vi "Array Manipulation.vi"() -> ()   [LabVIEW 2015]
doc: "This VI shows how different array functions can be used to manipulate data. There are also examples showing how we can use the Polymorphic functionality built into LabVIEW to easily modify the data in an array. \n\nExamine the different cases and read the comments on the block diagram for more details"
uses:
  <vilib>/measure/NI_MABase.lvlib
panel:
  in  "Stop Button":bool
  in  "Tab Control":T1(tab)
  out "Concatenated Data Array":dbl[](array[numeric])
  out "Concatenated Data":dbl[](graph)
  in  "Subtract?":bool
  out "Add or Subtract Data Array":dbl[](array[numeric])
  out "Add or Subtract Data":dbl[](graph)
  in  "Select Channel":u16(ring) items=["Channel 0", "Channel 1"]
  out "Single Channel of Data Array":dbl[](array[numeric])
  out "Single Channel of Data":dbl[](graph)
  out "Size of Array":i32
  in  "Offset":dbl(slide)=-8.326672684688674e-17 scale=-5.0..5.0
  out "Waveform Data":waveform(dbl)[](graph)
  out "Data Channel Array":dbl[][](array[numeric])
  in  "Channel 1 Offset":dbl(slide)=-8.326672684688674e-17 scale=-5.0..5.0
  out "All Data Channel":dbl[][](graph)
  out "Size of Array":i32[](array[numeric])
  out "Subset Data Array":dbl[][](array[numeric])
  in  "Start Value":i32(slide)=10 scale=0.0..1000.0
  out "Subset Data":dbl[][](graph)
  in  "Length":i32(slide)=1000 scale=0.0..1000.0
  # "Rows"
  # "Columns"
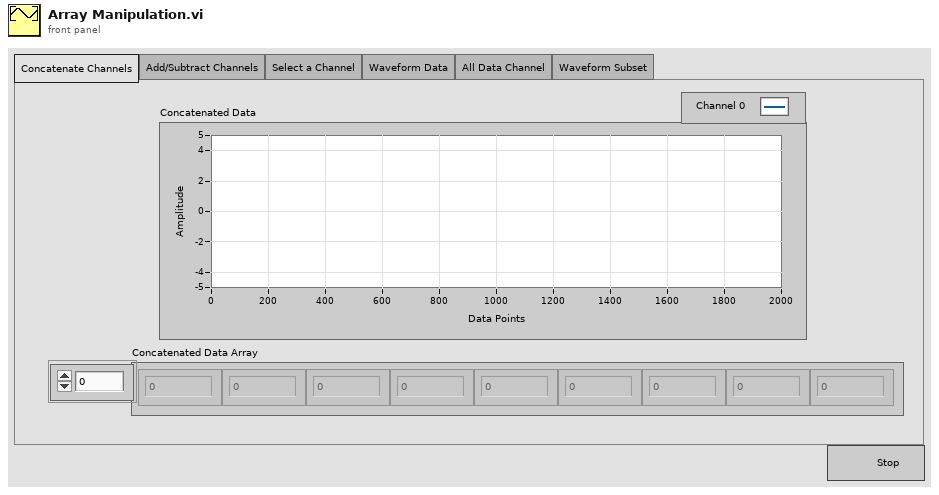
[diagram p1: front panel]
types:
  T1 = enum32{"Concatenate Channels", "Add/Subtract Channels", "Select a Channel", "Waveform Data", "All Data Channel", "Waveform Subset"}
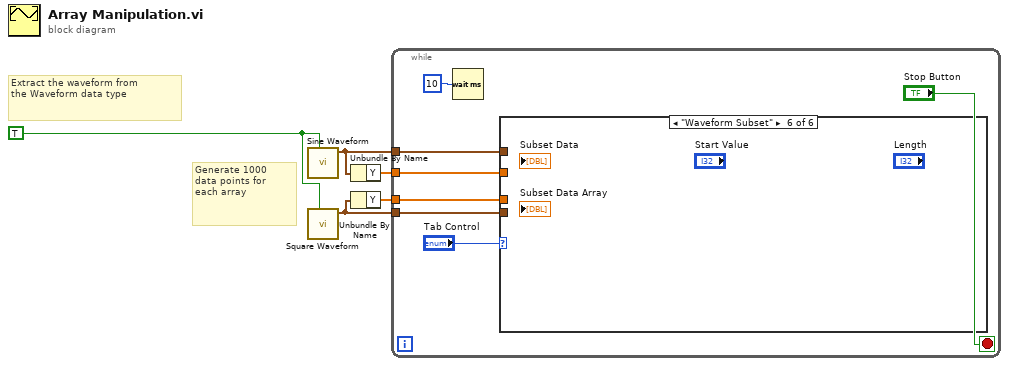
[diagram p0: block diagram]
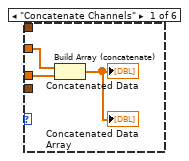
[diagram p2: hidden frame]
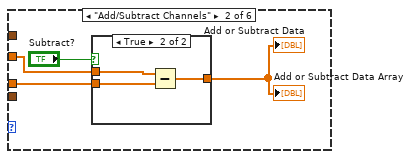
[diagram p3: hidden frame]
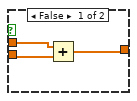
[diagram p4: hidden frame]
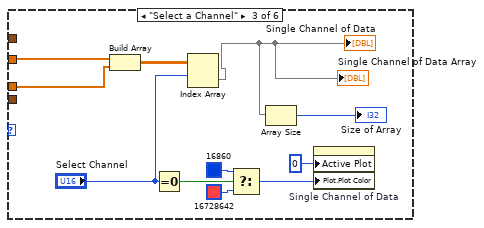
[diagram p5: hidden frame]
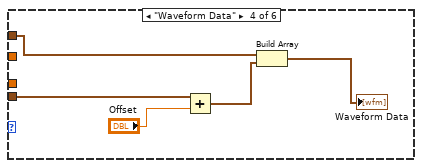
[diagram p6: hidden frame]
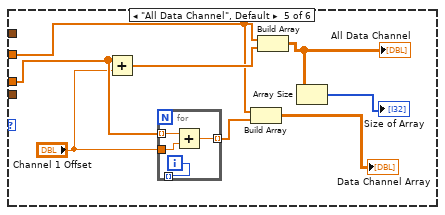
[diagram p7: hidden frame]
diagram:
  w5 = TRUE
  # "Extract the waveform from \nthe Waveform data type"
  # "Generate 1000\ndata points for \neach array"
  n1 = call <vilib>:"Sine Waveform.vi"("reset signal"=w5) -> ("signal out"=w2:waveform(dbl))  [unwired: 9 in, 1 out]
  n2 = call <vilib>:"Square Waveform.vi"("reset signal"=w5) -> ("signal out"=w1:waveform(dbl))  [unwired: 9 in, 1 out]
  n3 = Unbundle By Name(w2) -> ("Y"=w4:dbl[])
  n4 = Unbundle By Name(w1) -> ("Y"=w3:dbl[])
  n5 = while {
    tunnel: w4 -> [w10]
    tunnel: w3 -> [w9]
    tunnel: w2 -> [w8]
    tunnel: w1 -> [w7]
    stop <- "Stop Button" stop-if-true
    n6 = Wait (ms)(milliseconds to wait=u32 10) -> ()  [unwired: 1 out]
    n7 = case shown="\"Waveform Subset\"" "Tab Control" {
      tunnel: w10 -> [w15 w19 w31 _ w42 _]
      tunnel: w9 -> [w14 w18 w30 _ w48 _]
      tunnel: w8 -> [_ _ _ w40 _ _]
      tunnel: w7 -> [_ _ _ w39 _ _]
      frame "Concatenate Channels" {
        n8 = Build Array (concatenate)(w15, w14) -> (→"Concatenated Data" →"Concatenated Data Array":dbl[])
      }
      frame "Add/Subtract Channels" {
        n9 = case shown="True" "Subtract?" {
          tunnel: w19 -> [w22 w25]
          tunnel: w18 -> [w21 w24]
          tunnel: [w20 w23] -> w17
          frame False {
            n10 = Add(x=w22, y=w21) -> (x+y=w20:dbl[])
          }
          frame True {
            n11 = Subtract(x=w25, y=w24) -> (x-y=w23:dbl[])
          }
        }
        "Add or Subtract Data" <- w17
        "Add or Subtract Data Array" <- w17
      }
      frame "Select a Channel" {
        n12 = Build Array(w31, w30) -> (w29:dbl[][])
        n13 = Equal To 0?(x="Select Channel") -> (x = 0?=w32:bool)
        n14 = Index Array(array=w29, index (row)="Select Channel") -> (element=w27:dbl[])  [unwired: 1 in]
        "Single Channel of Data" <- w27
        "Single Channel of Data Array" <- w27
        n15 = Select(t=u32 16860, s=w32, f=u32 16728642) -> (s? t:f=w35:u32)
        n16 = Array Size(array=w27) -> (size(s)=→"Size of Array":i32)
        n17 = property on="Single Channel of Data" class="WFGraph (strict)"("Active Plot"=u32 0, "Plot.Plot Color"=w35) -> ()  [unwired: 2 in, 2 out]
      }
      frame "Waveform Data" {
        n18 = Add(x=w39, y="Offset") -> (x+y=w37:waveform(dbl))
        n19 = Build Array(w40, w37) -> (→"Waveform Data":waveform(dbl)[])
      }
      frame "All Data Channel", Default {
        n20 = Add(x=w48, y="Channel 1 Offset") -> (x+y=w49:dbl[])
        n21 = for {
          tunnel: w48 -> [w53] mode=indexing
          tunnel: [w51] -> _ mode=indexing
          tunnel: "Channel 1 Offset" -> [w52]
          tunnel: [w50] -> w46 mode=indexing
          i -> [w51]
          n22 = Add(x=w53, y=w52) -> (x+y=w50:dbl)
        }
        n23 = Build Array(w42, w46) -> (→"Data Channel Array":dbl[][])
        n24 = Build Array(w42, w49) -> (w43:dbl[][])
        "All Data Channel" <- w43
        n25 = Array Size(array=w43) -> (size(s)=→"Size of Array":i32[])
      }
      frame "Waveform Subset" {
      }
    }
  }
